vi "14 benched.vi"() -> ()   [LabVIEW 2021]
uses:
  <vilib>/Analysis/baseanly.llb/Mean (DBL).vi
  <vilib>/Analysis/NI_AALBase.lvlib
panel:
  out "mean_exec_time (sec)":dbl format="%0.6f"
  out "max index(es)":i32
  in  "n_Collatz":i32=1000000 min=1 step=1
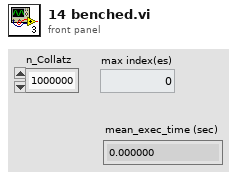
[diagram p1: front panel]
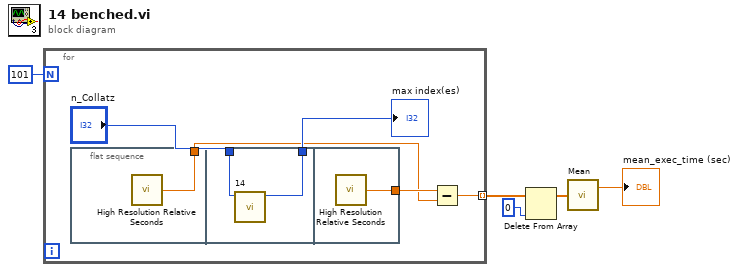
[diagram p0: block diagram]
diagram:
  n1 = for {
    N: 101 -> [_]
    tunnel: [w6] -> w5 mode=indexing
    n2 = flat-sequence {
      tunnel: [w11] -> w7
      tunnel: "n_Collatz" -> [w13]
      tunnel: [w12] -> w10
      tunnel: [w14] -> w8
      frame #0 {
        n3 = call <vilib>:"High Resolution Relative Seconds.vi"() -> ("relative seconds"=w11:dbl)
      }
      frame #1 {
        n4 = call "14.vi"("n_Collatz"=w13) -> ("max index(es)"=w12:i32)  [unwired: 10 in]
      }
      frame #2 {
        n5 = call <vilib>:"High Resolution Relative Seconds.vi"() -> ("relative seconds"=w14:dbl)
      }
    }
    n6 = Subtract(x=w8, y=w7) -> (x-y=w6:dbl)
    "max index(es)" <- w10
  }
  n7 = Delete From Array(array=w5, index=0) -> (array with subset deleted=w3:dbl[])  [unwired: 1 in, 1 out]
  n8 = call-poly <vilib>:"Mean.vi"("X"=w3) -> ("mean"=→"mean_exec_time (sec)":dbl)  [unwired: 1 out]
